vi "dfd_Group Delay_Error Vector.vi"(10 "Coefficients":cluster{"r":dbl[], "theta":dbl[], "offset":dbl}, 11 "Design Info":T1={"p"=2, "freq grid"=[], "d"=[], "weight"=[], "Order"=0, "radius"=0.0}) -> (1 "Error":dbl[](array[numeric]), 2 "Coefficients (dup)":cluster{"r":dbl[], "theta":dbl[], "offset":dbl}, 3 "Design Info (dup)":T1={"p"=2, "freq grid"=[], "d"=[], "weight"=[], "Order"=0, "radius"=0.0})   [LabVIEW 2017, in "NI_DigFilter_Design.lvlib"]
uses:
  <vilib>/addons/Digital Filter Design/NI_DigFilter_Design.lvlib
  <vilib>/addons/Digital Filter Design/_GroupDelay.llb/dfd_Group Delay_Design Info.ctl
  <vilib>/Analysis/baseanly.llb/Real A x B.vi
  <vilib>/Analysis/NI_AALBase.lvlib
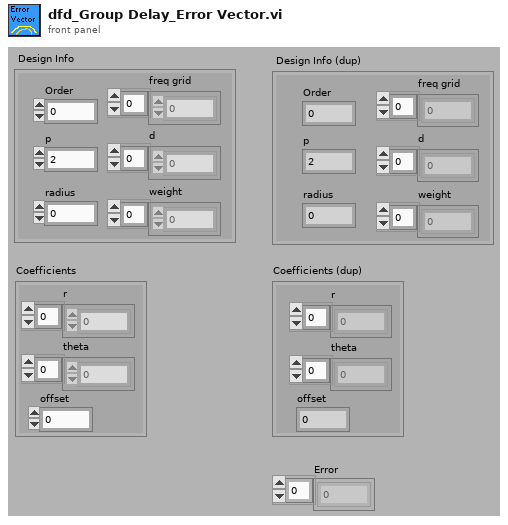
[diagram p1: front panel]
types:
  T1 = typedef "dfd_Group Delay_Design Info.ctl" = cluster{"p":i32, "freq grid":dbl[], "d":dbl[], "weight":dbl[], "Order":i32, "radius":dbl}
  T2 = typedef "NI_Matrix.lvlib/RealMatrix.ctl" = dbl[][]
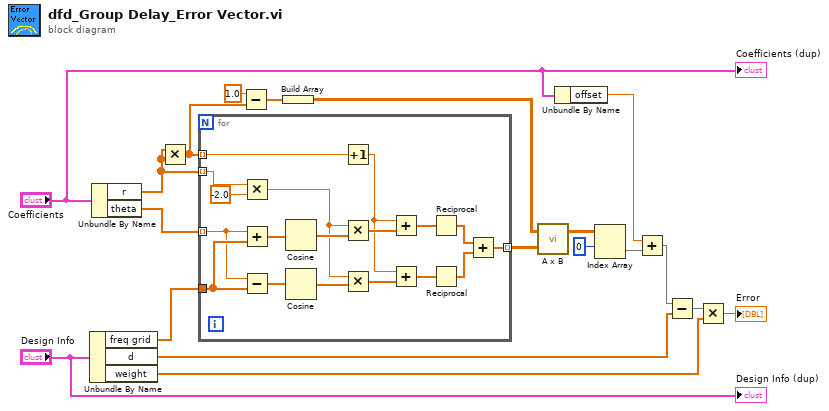
[diagram p0: block diagram]
diagram:
  n1 = Unbundle By Name("Design Info") -> ("freq grid"=w13:dbl[], "d"=w12:dbl[], "weight"=w9:dbl[])
  n2 = Unbundle By Name("Coefficients") -> ("r"=w8:dbl[], "theta"=w14:dbl[])
  n3 = Multiply(x=w8, y=w8) -> (x*y=w7:dbl[])
  n4 = for {
    tunnel: w8 -> [w33] mode=indexing
    tunnel: w14 -> [w36] mode=indexing
    tunnel: w13 -> [w37]
    tunnel: [w22] -> w18 mode=indexing
    tunnel: w7 -> [w21] mode=indexing
    n5 = Multiply(x=w33, y=-2.0) -> (x*y=w20:dbl)
    n6 = Add(x=w36, y=w37) -> (x+y=w34:dbl[])
    n7 = Subtract(x=w36, y=w37) -> (x-y=w35:dbl[])
    n8 = Cosine(x=w34) -> (cos(x)=w30:dbl[])
    n9 = Cosine(x=w35) -> (cos(x)=w31:dbl[])
    n10 = Increment(x=w21) -> (x+1=w27:dbl)
    n11 = Multiply(x=w20, y=w30) -> (x*y=w28:dbl[])
    n12 = Multiply(x=w20, y=w31) -> (x*y=w29:dbl[])
    n13 = Add(x=w27, y=w28) -> (x+y=w25:dbl[])
    n14 = Add(x=w27, y=w29) -> (x+y=w26:dbl[])
    n15 = Reciprocal(x=w25) -> (1/x=w24:dbl[])
    n16 = Reciprocal(x=w26) -> (1/x=w23:dbl[])
    n17 = Add(x=w24, y=w23) -> (x+y=w22:dbl[])
  }
  n18 = Subtract(x=1.0, y=w7) -> (x-y=w5:dbl[])
  n19 = Build Array(w5) -> (w4:dbl[][])
  n20 = call-poly <vilib>:"A x B.vi"("B"=w18, "A"=w4) -> ("A x B"=w17:T2)  [unwired: 1 out]
  n21 = Unbundle By Name("Coefficients") -> ("offset"=w3:dbl)
  n22 = Index Array(array=w17, index (row)=0) -> (element=w10:dbl[])  [unwired: 1 in]
  n23 = Add(x=w3, y=w10) -> (x+y=w11:dbl[])
  n24 = Subtract(x=w11, y=w12) -> (x-y=w15:dbl[])
  n25 = Multiply(x=w15, y=w9) -> (x*y=→"Error":dbl[])
  "Design Info (dup)" <- "Design Info"
  "Coefficients (dup)" <- "Coefficients"
